vi "Multiple Chassis Synchronization - Scopes Synchronized without TCLK.vi"() -> ()   [LabVIEW 2026]
uses:
  SubVIs/NI SYNC Abstraction/Lib/Clock Routing.ctl
  <instrlib>/niScope/Controls/niScope export destinations.ctl
  SubVIs/NI SYNC Abstraction/Lib/Trigger Routing.ctl
  Types/MyState.ctl
  <instrlib>/niScope/Controls/niScope input clock source.ctl
  Types/MyVariables.ctl
  <instrlib>/niScope/Controls/niScope exportable signals.ctl
  <instrlib>/niFgen/niFgen.llb/niFgen Output Mode.ctl
  <instrlib>/niScope/Configure/Trigger/niScope Configure Trigger Edge.vi
  <instrlib>/niScope/Configure/Trigger/niScope Configure Trigger Digital.vi
  <instrlib>/niSync/niSync.llb/niSync Initialize (IVI).vi
  SubVIs/NI SYNC Abstraction/Lib/Connect Clock Terminals-Array.vi
  SubVIs/NI SYNC Abstraction/Lib/Connect Clock Terminals.vi
  SubVIs/NI SYNC Abstraction/Lib/Connect Trigger Terminals.vi
  <instrlib>/niScope/Acquire/Fetch/niScope Fetch Cluster.vi
  SubVIs/NI SYNC Abstraction/Lib/Disonnect Trigger Terminals.vi
  SubVIs/NI SYNC Abstraction/Lib/Disconnect Clock Terminals-Array.vi
  SubVIs/NI SYNC Abstraction/Lib/Disconnect Clock Terminals.vi
panel:
  in  "Tab Control":T1(tab)
  in  "Master.Scope":refnum<k15>="PXI1_SCOPE1"
  in  "Rest.Scopes":refnum<k15>[](array[refnum])=["PXI2_SCOPE2"]
  in  "Master.6674T_1":refnum<k15>="PXI1_MasterSync"
  in  "Rest.6674T_1":refnum<k15>="PXI2_SlaveSync"
  in  "FGEN.Ref":refnum<k15>="PXI1_FGEN1"
  in  "Routing":enum32{"Clock Routing", "Reference Trigger"}(tab)
  in  "Rest.In --> Clk10":T2={"Source Terminal"="ClkIn", "Destination Terminal"="PXI_Clk10_In"}
  in  "Master.In --> Clk10":T2={"Source Terminal"="ClkIn", "Destination Terminal"="PXI_Clk10_In"}
  in  "Master.Clock --> Out":T2={"Source Terminal"="Oscillator", "Destination Terminal"="ClkOut"}
  in  "Rest.Ref Trigger Source":T3="VAL_RTSI_0"
  in  "Rest.PFI --> Ref Trigger":T4={"Source"="PFI0", "Destination"="PXI_Trig0", "Synchronization Clock"="SyncClkAsync"}
  in  "Master.Ref Trigger --> PFI":T4={"Source"="PXI_Trig0", "Destination"="PFI0", "Synchronization Clock"="SyncClkAsync"}
  in  "Master.Ref Trigger Export":T3="VAL_RTSI_0"
  out "Waveform Graph":T5(graph)
  out "Sample Offset":dbl
  out "error out":errorcluster
  out "Offset Time (s)":dbl format="%#_p"
  # "Scope"
  # "Sync"
  # "Master"
  # "Ref Trigger Export"
  # "None"
  # "None"
  # "None"
  # "Sync"
  # "Scope"
  # "Rest"
  # "Ref Trigger Source"
  # "None"
  # "None"
  # "None"
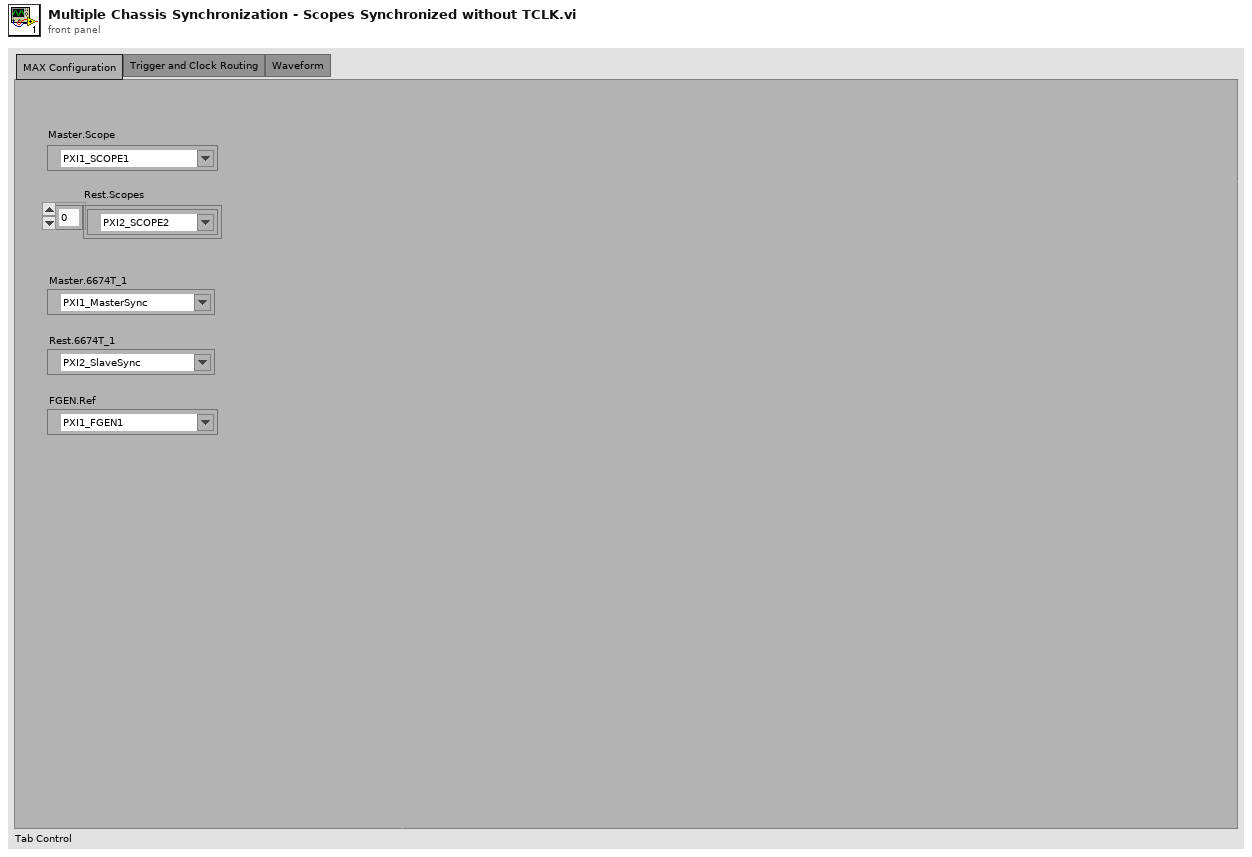
[diagram p1: front panel]
types:
  T1 = enum32{"MAX Configuration", "Trigger and Clock Routing", "Waveform"}
  T2 = typedef "Clock Routing.ctl" = cluster{"Source Terminal":string, "Destination Terminal":string}
  T3 = typedef "niScope export destinations.ctl" = string
  T4 = typedef "Trigger Routing.ctl" = cluster{"Source":string, "Destination":string, "Synchronization Clock":string}
  T5 = cluster{"relativeInitialX":dbl, "xIncrement":dbl, "wfm":dbl[]}[]
  T6 = typedef "niScope input clock source.ctl" = u16
  T7 = typedef "MyState.ctl" = enum16{"Initialize", "SCOPE: Config.Master", "SCOPE: Config.Rest", "SYNC: Device.Init", "SYNC: ConnectClock.Master", "SYNC: ConnectClock.Rest", "SYNC: ConnectSyncPulse.Master", "SYNC: ConnectSyncPulse.Rest", "SYNC: ConnectRefTrigger.Master", "SYNC: ConnectRefTrigger.Rest", "TCLK: Config.Master", "TCLK: Config.Rest", "TCLK: ApplyManualCalibration", "TCLK: SendSyncPulse", "SYNC: DisconnectSyncPulse.Master", "SYNC: DisconnectSyncPulse.Rest", "SYNC: ConnectStartTrigger.Master", "SYNC: ConnectStartTrigger.Rest", "TCLK: Commit", "FGEN: StartSquareWave", "SCOPE: Acquire", "FGEN: StopSquareWave", "SYNC: DisconnectStartTrigger.Master", "SYNC: DisconnectStartTrigger.Rest", "SYNC: DisconnectRefTrigger.Master", "SYNC: DisconnectRefTrigger.Rest", "SYNC: DisconnectClock.Master", "SYNC: DisconnectClock.Rest", "Shutdown"}
  T8 = typedef "MyVariables.ctl" = cluster{"Master":cluster{"TimeSync.Ref":refnum<k15>, "TCLK.Ref":refnum<k20>, "Clock":cluster{"Clock --> Out":T2, "In --> Clk10":T2}, "Sync Pulse":cluster{"Sync Pulse Export":string, "Sync Pulse Export --> PFI":T4, "PFI --> Sync Pulse Source":T4, "Sync Pulse Source":string}, "Start Trigger":cluster{"Start Trigger Export":T3, "Start Trigger --> PFI":T4}, "Scope.Ref":refnum<k15>, "Ref Trigger":cluster{"Ref Trigger Export":T3, "Ref Trigger --> PFI":T4}}, "Rest":cluster{"TimeSync.Ref":refnum<k15>, "TCLK.Refs":refnum<k20>[], "Clock":cluster{"In --> Clk10":T2}, "Sync Pulse":cluster{"PFI --> Sync Pulse Source":T4, "Sync Pulse Source":string}, "Start Trigger":cluster{"PFI --> Start Trigger":T4, "Start Trigger Source":T3}, "Scope.Refs":refnum<k15>[], "Ref Trigger":cluster{"PFI --> Ref Trigger":T4, "Ref Trigger Source":T3}}, "FGEN.Ref":refnum<k15>}
  T9 = typedef "niScope exportable signals.ctl" = u16
  T10 = typedef "niFgen Output Mode.ctl" = u32
  T11 = cluster{"relativeInitialX":dbl, "xIncrement":dbl, "wfm":dbl[]}
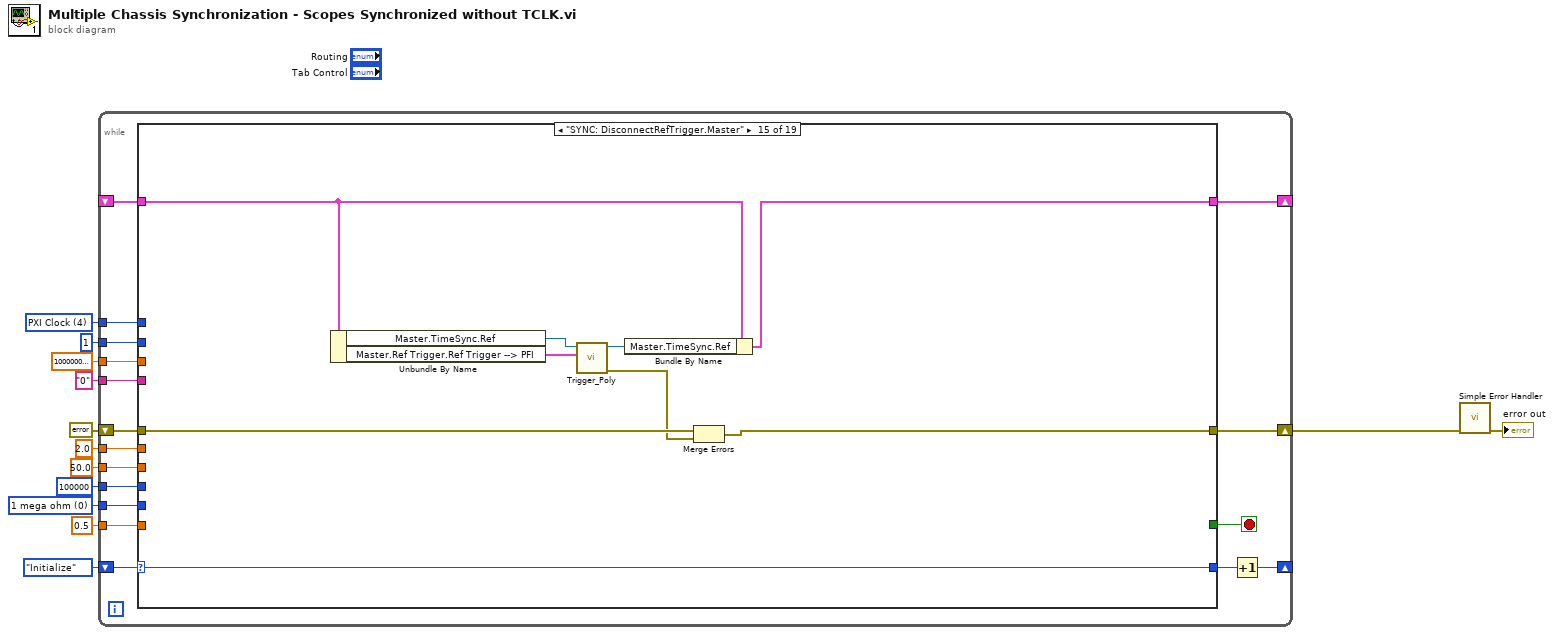
[diagram p0: block diagram]
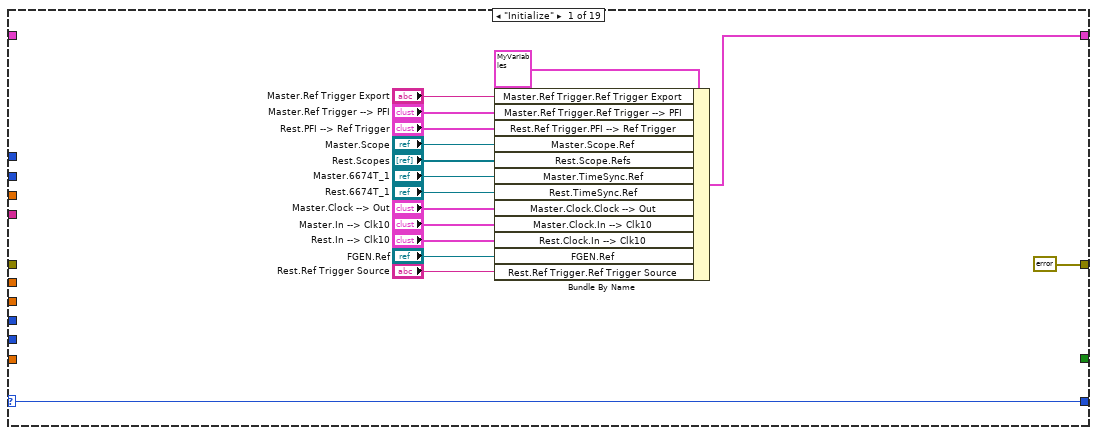
[diagram p2: hidden frame]
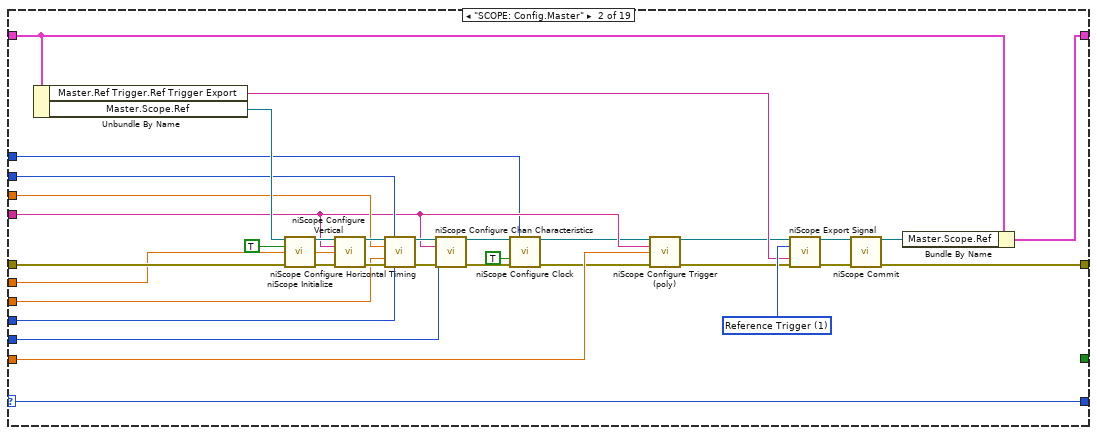
[diagram p3: hidden frame]
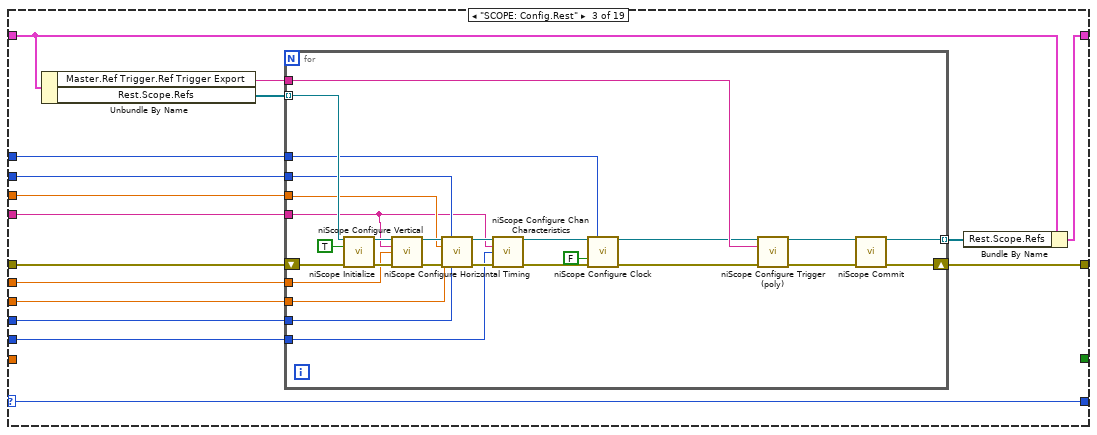
[diagram p4: hidden frame]
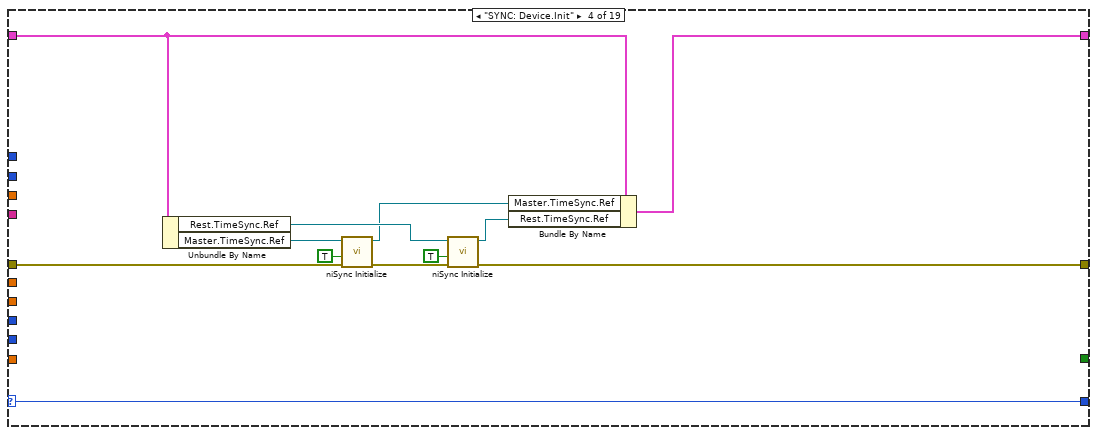
[diagram p5: hidden frame]
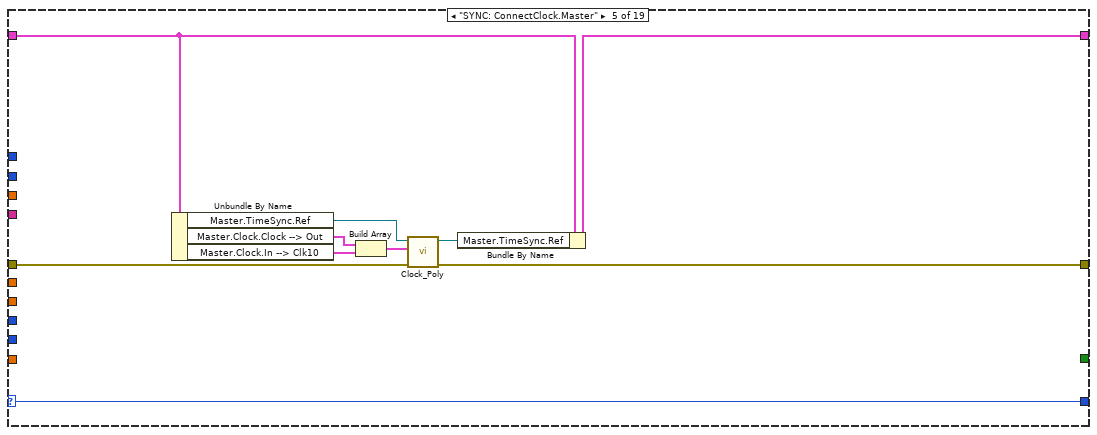
[diagram p6: hidden frame]
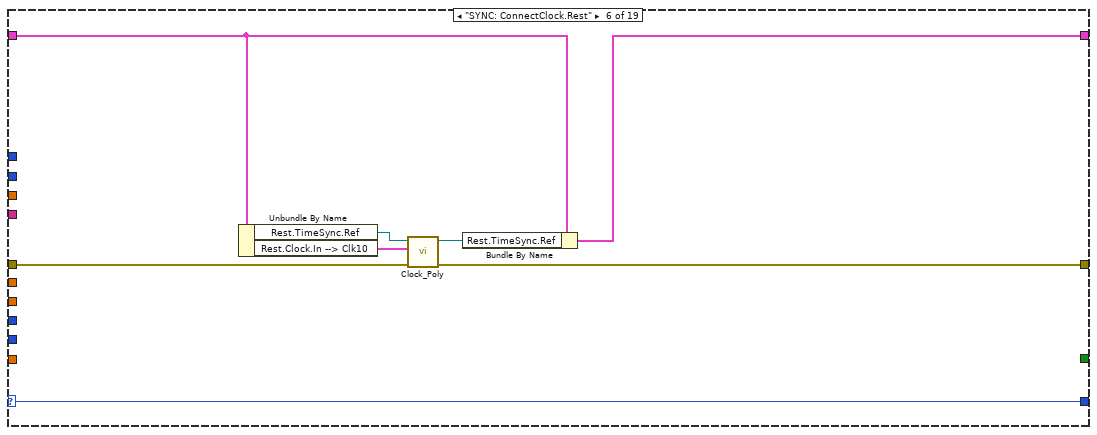
[diagram p7: hidden frame]
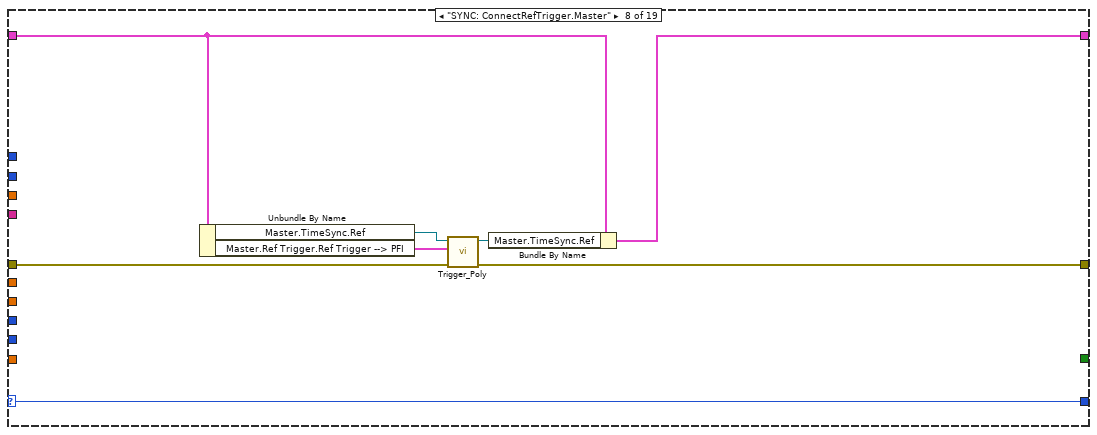
[diagram p9: hidden frame]
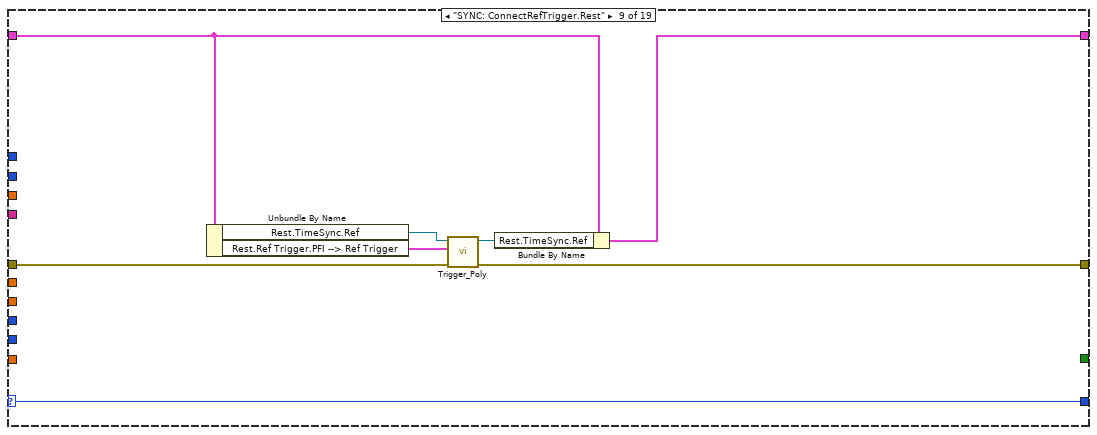
[diagram p10: hidden frame]
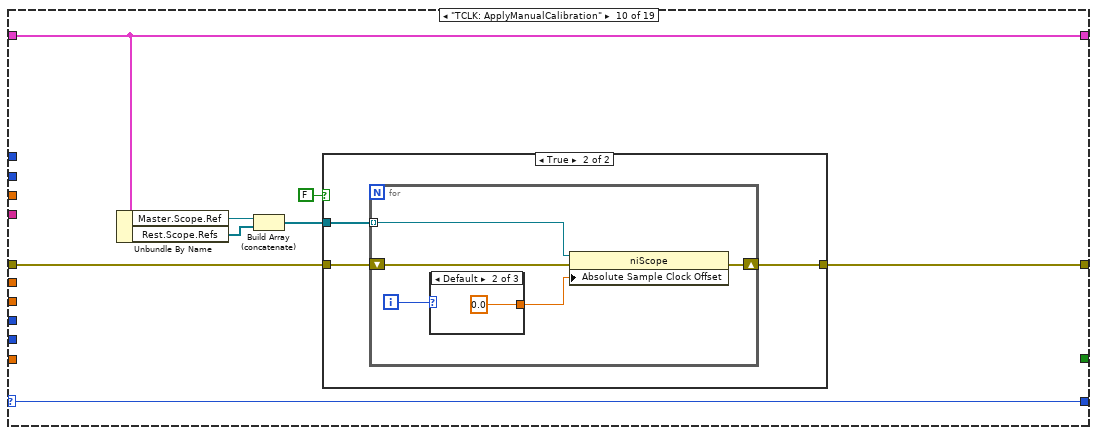
[diagram p11: hidden frame]
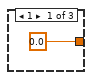
[diagram p13: hidden frame]
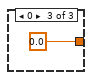
[diagram p14: hidden frame]
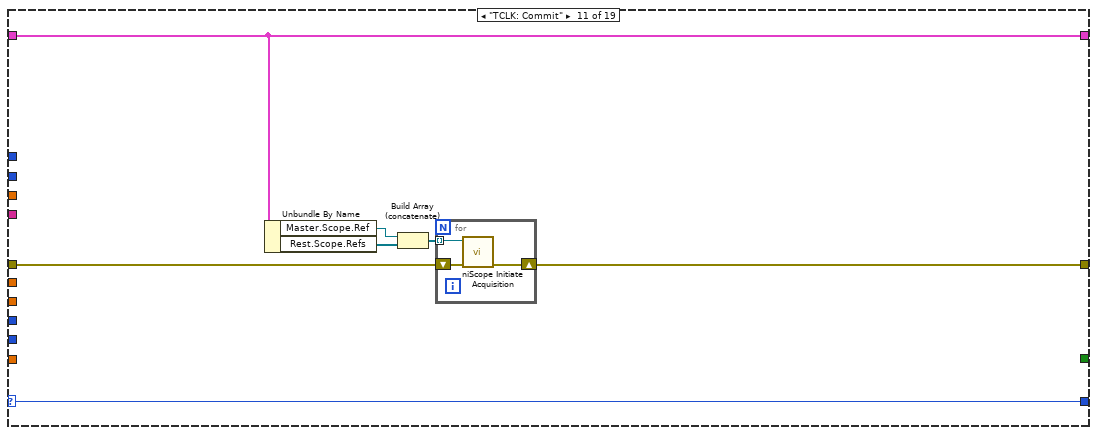
[diagram p15: hidden frame]
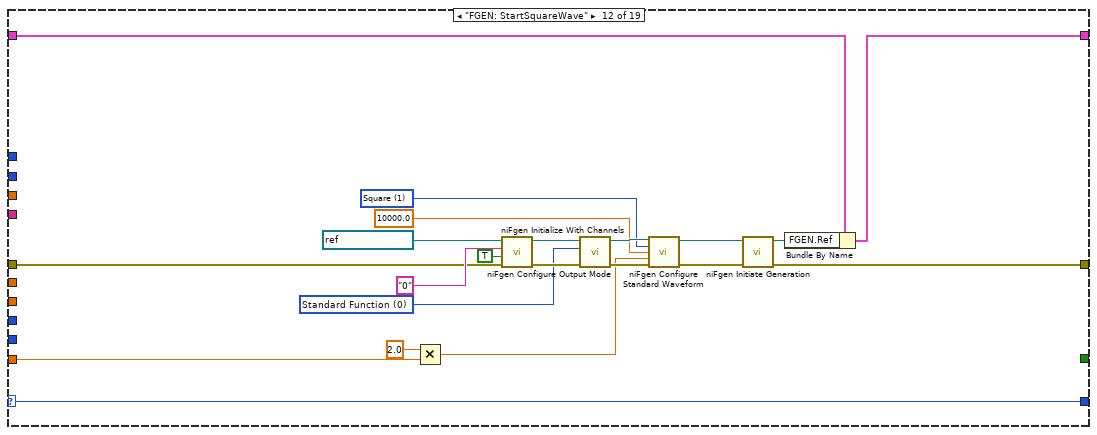
[diagram p16: hidden frame]
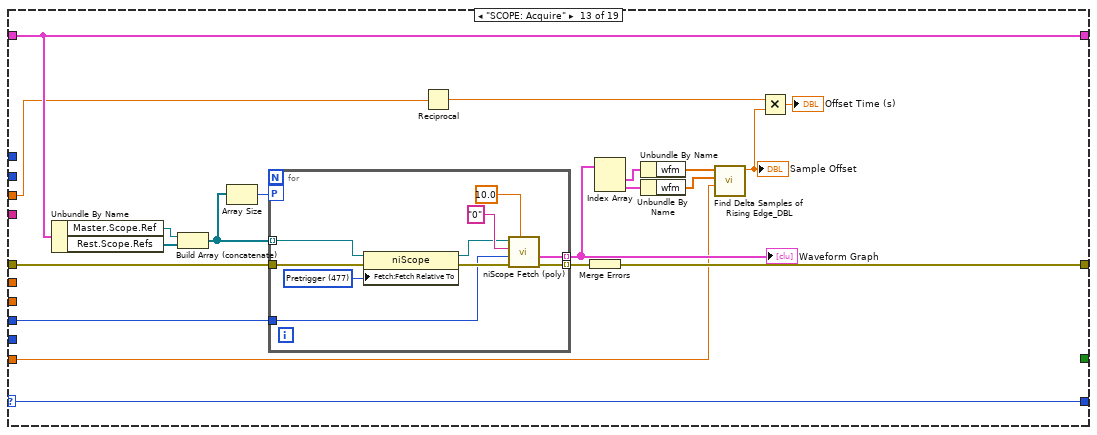
[diagram p17: hidden frame]
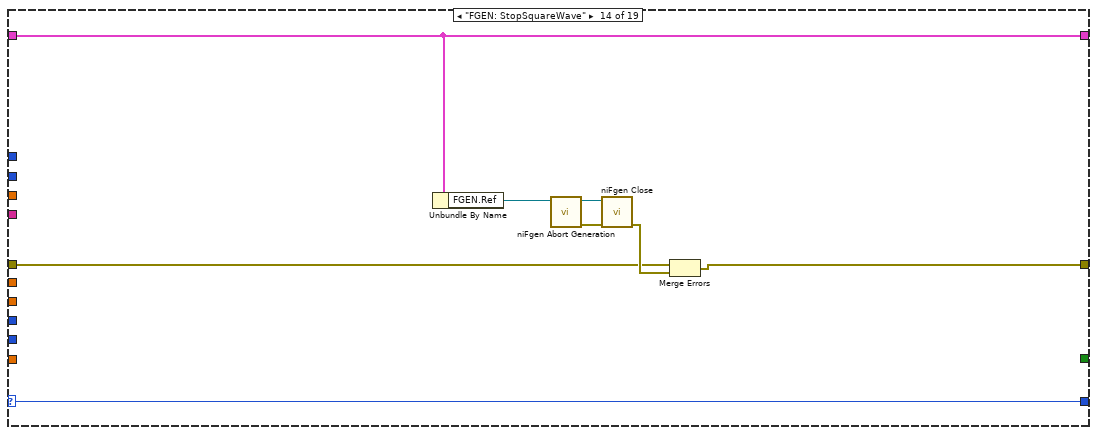
[diagram p18: hidden frame]
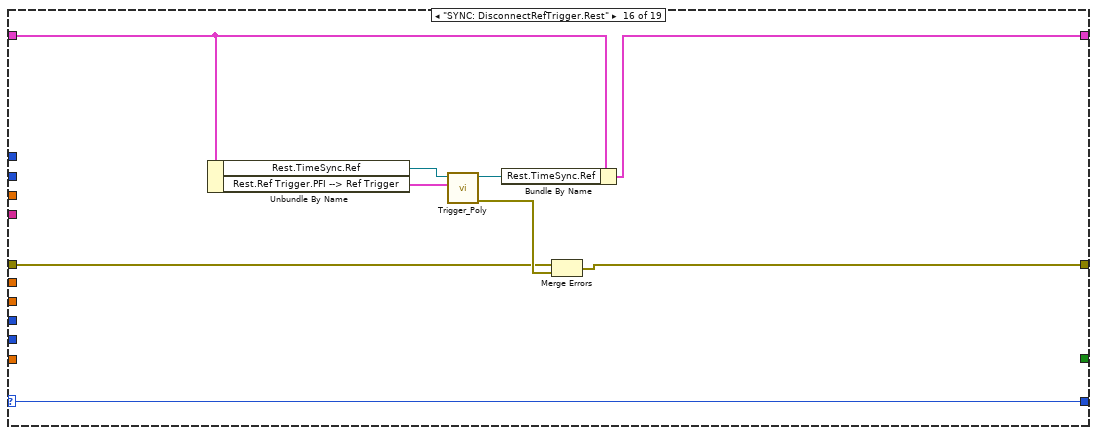
[diagram p19: hidden frame]
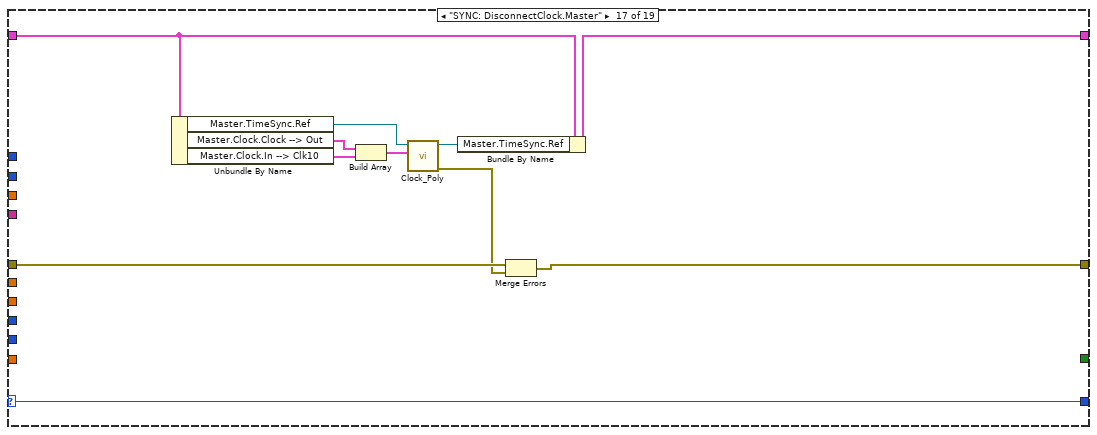
[diagram p20: hidden frame]
diagram:
  w1 = T6 4 items=["None"=0, "RTSI Clock"=1, "PFI 0"=6, "PFI 1"=2, "PFI 2"=3, "PXI Clock"=4, "External"=5, "Clock In"=7] ("input clock source")
  w5 = u32 0 items=["1 mega ohm"=0, "50 ohms"=2] ("input impedance")
  n1 = while {
    shift-right: [w23] -> _
    shift-left: MyState."Initialize" -> [w30]
    shift-right: [w29] -> _
    shift-left: _ -> [w28]
    shift-right: [w26] -> w11
    shift-left: errorcluster {"status"=FALSE, "code"=0, "source"=""} ("error out") -> [w27]
    tunnel: 100000000.0 ("min sample rate") -> [w22]
    tunnel: 100000 ("min record length") -> [w21]
    tunnel: 2.0 ("vertical offset") -> [w20]
    tunnel: 50.0 ("reference position") -> [w19]
    tunnel: w5 -> [w18]
    tunnel: 1 ("number of records") -> [w17]
    tunnel: "0" ("channels") -> [w16]
    tunnel: 0.5 ("trigger level") -> [w15]
    tunnel: w1 -> [w14]
    stop <- w24 stop-if-true
    n2 = case shown="\"SYNC: DisconnectRefTrigger.Master\"" w30 {
      selector: w30 -> [w39 w80 w96 w125 w136 w147 w156 w158 w166 w180 w199 w210 w243 w254 w266 w275 w283 w295 w301]
      tunnel: [w40 w79 w95 w129 w144 w152 w154 w163 w171 w179 w196 w207 w240 w259 w269 w278 w289 w298 w312] -> w29
      tunnel: w28 -> [_ w70 w92 w130 w145 w153 w154 w164 w172 w179 w196 w209 w240 w259 w270 w279 w290 w299 w312]
      tunnel: [w39 w80 w96 w125 w136 w147 w156 w158 w166 w180 w199 w210 w243 w254 w266 w275 w283 w295 w301] -> w25
      tunnel: [errorcluster {"status"=FALSE, "code"=0, "source"=""} ("error out") w56 w94 w126 w141 w149 w155 w160 w168 w174 w194 w211 w237 w255 w262 w272 w281 w292 w302] -> w26
      tunnel: w27 -> [_ w71 w93 w124 w137 w148 w155 w159 w167 w175 w195 w212 w242 w256 w264 w271 w282 w293 w305]
      tunnel: [_ _ _ _ _ _ _ _ _ _ _ _ _ _ _ _ _ _ TRUE] -> w24
      tunnel: w22 -> [_ w64 w87 _ _ _ _ _ _ _ _ _ w228 _ _ _ _ _ _]
      tunnel: w21 -> [_ w63 w83 _ _ _ _ _ _ _ _ _ w229 _ _ _ _ _ _]
      tunnel: w20 -> [_ w62 w85 _ _ _ _ _ _ _ _ _ _ _ _ _ _ _ _]
      tunnel: w19 -> [_ w61 w84 _ _ _ _ _ _ _ _ _ _ _ _ _ _ _ _]
      tunnel: w18 -> [_ w60 w82 _ _ _ _ _ _ _ _ _ _ _ _ _ _ _ _]
      tunnel: w17 -> [_ w59 w88 _ _ _ _ _ _ _ _ _ _ _ _ _ _ _ _]
      tunnel: w16 -> [_ w58 w86 _ _ _ _ _ _ _ _ _ _ _ _ _ _ _ _]
      tunnel: w15 -> [_ w57 _ _ _ _ _ _ _ _ _ w205 w224 _ _ _ _ _ _]
      tunnel: w14 -> [_ w47 w81 _ _ _ _ _ _ _ _ _ _ _ _ _ _ _ _]
      frame "Initialize" {
        n3 = Bundle By Name(cluster=T8 {"Master"={"TimeSync.Ref"="PXI_Trig0", "TCLK.Ref"=refnum, "Clock"={"Clock --> Out"={"Source Terminal"="Oscillator", "Destination Terminal"="ClkOut"}, "In --> Clk10"={"Source Terminal"="ClkIn", "Destination Terminal"="PXI_Clk10_In"}}, "Sync Pulse"={"Sync Pulse Export"="SyncClkFullSpeed", "Sync Pulse Export --> PFI"={"Source"="ClkIn", "Destination"="PXI_Clk10_In", "Synchronization Clock"="SyncClkAsync"}, "PFI --> Sync Pulse Source"={"Source"="PXI_Trig2", "Destination"="PFI2", "Synchronization Clock"="SyncClkAsync"}, "Sync Pulse Source"="PFI1"}, "Start Trigger"={"Start Trigger Export"="PXI_Trig2", "Start Trigger --> PFI"={"Source"="SyncClkAsync", "Destination"="VAL_RTSI_2", "Synchronization Clock"=""}}, "Scope.Ref"="", "Ref Trigger"={"Ref Trigger Export"="VAL_RTSI_2", "Ref Trigger --> PFI"={"Source"="PXI_Trig3", "Destination"="PFI0", "Synchronization Clock"="SyncClkAsync"}}}, "Rest"={"TimeSync.Ref"="", "TCLK.Refs"=[], "Clock"={"In --> Clk10"={"Source Terminal"="PXI_Trig0", "Destination Terminal"="PFI2"}}, "Sync Pulse"={"PFI --> Sync Pulse Source"={"Source"="PFI1", "Destination"="PXI_Trig1", "Synchronization Clock"="SyncClkAsync"}, "Sync Pulse Source"="PXI_Trig1"}, "Start Trigger"={"PFI --> Start Trigger"={"Source"="PFI1", "Destination"="PXI_Trig2", "Synchronization Clock"="SyncClkAsync"}, "Start Trigger Source"="VAL_RTSI_2"}, "Scope.Refs"=[], "Ref Trigger"={"PFI --> Ref Trigger"={"Source"="PFI0", "Destination"="PXI_Trig3", "Synchronization Clock"="SyncClkAsync"}, "Ref Trigger Source"="VAL_RTSI_3"}}, "FGEN.Ref"=""} ("Routes"), "Master.Ref Trigger.Ref Trigger Export"="Master.Ref Trigger Export", "Master.Ref Trigger.Ref Trigger --> PFI"="Master.Ref Trigger --> PFI", "Rest.Ref Trigger.PFI --> Ref Trigger"="Rest.PFI --> Ref Trigger", "Master.Scope.Ref"="Master.Scope", "Rest.Scope.Refs"="Rest.Scopes", "Master.TimeSync.Ref"="Master.6674T_1", "Rest.TimeSync.Ref"="Rest.6674T_1", "Master.Clock.Clock --> Out"="Master.Clock --> Out", "Master.Clock.In --> Clk10"="Master.In --> Clk10", "Rest.Clock.In --> Clk10"="Rest.In --> Clk10", "FGEN.Ref"="FGEN.Ref", "Rest.Ref Trigger.Ref Trigger Source"="Rest.Ref Trigger Source") -> (w40:T8)
      }
      frame "SCOPE: Config.Master" {
        w66 = T9 1 items=["None"=0, "Start Trigger"=2, "Advance Trigger"=5, "Reference Trigger"=1, "End of Record Event"=4, "End of Acquisition Event"=3, "Ready for Start Event"=7, "Ready for Advance Event"=6, "Ready for Reference Event"=10, "Reference Clock"=100, "Sample Clock"=101, "5 Volt Power"=13] ("signal")
        n4 = Unbundle By Name(w70) -> ("Master.Ref Trigger.Ref Trigger Export"=w65:T3, "Master.Scope.Ref"=w69:refnum<k15>)
        n5 = call <instrlib>:"niScope Initialize.vi"("resource name"=w69, "id query"=TRUE, "error in"=w71) -> ("instrument handle"=w77:refnum<k15>, "error out"=w74:errorcluster)  [unwired: 11 in]
        n6 = call <instrlib>:"niScope Configure Vertical.vi"("instrument handle"=w77, "channels"=w58, "vertical range"=w62, "error in"=w74) -> ("instrument handle out"=w76:refnum<k15>, "error out"=w73:errorcluster)  [unwired: 10 in]
        n7 = call <instrlib>:"niScope Configure Horizontal Timing.vi"("instrument handle"=w76, "number of records"=w59, "min sample rate"=w64, "reference position"=w61, "error in"=w73, "min record length"=w63) -> ("instrument handle out"=w75:refnum<k15>, "error out"=w72:errorcluster)  [unwired: 8 in]
        n8 = call <instrlib>:"niScope Configure Chan Characteristics.vi"("instrument handle"=w75, "channels"=w58, "input impedance"=w60, "error in"=w72) -> ("instrument handle out"=w49:refnum<k15>, "error out"=w51:errorcluster)  [unwired: 10 in]
        n9 = call <instrlib>:"niScope Configure Clock.vi"("instrument handle"=w49, "input clock source"=w47, "master enabled"=TRUE, "error in"=w51) -> ("instrument handle out"=w48:refnum<k15>, "error out"=w50:errorcluster)  [unwired: 10 in]
        n10 = call-poly <instrlib>:"niScope Configure Trigger (poly).vi"("instrument handle"=w48, "trigger source"=w58, "trigger level"=w57, "error in"=w50) -> ("instrument handle out"=w53:refnum<k15>, "error out"=w54:errorcluster)  [unwired: 10 in]
        n11 = call <instrlib>:"niScope Export Signal.vi"("instrument handle"=w53, "signal"=w66, "output terminal"=w65, "error in"=w54) -> ("instrument handle out"=w67:refnum<k15>, "error out"=w68:errorcluster)  [unwired: 10 in]
        n12 = call <instrlib>:"niScope Commit.vi"("instrument handle"=w67, "error in"=w68) -> ("instrument handle out"=w55:refnum<k15>, "error out"=w56:errorcluster)  [unwired: 12 in]
        n13 = Bundle By Name(cluster=w70, "Master.Scope.Ref"=w55) -> (w79:T8)
      }
      frame "SCOPE: Config.Rest" {
        n14 = Unbundle By Name(w92) -> ("Master.Ref Trigger.Ref Trigger Export"=w89:T3, "Rest.Scope.Refs"=w90:refnum<k15>[])
        n15 = for {
          shift-right: [w104] -> w94
          shift-left: w93 -> [w116]
          tunnel: [w103] -> w91 mode=indexing
          tunnel: w90 -> [w113] mode=indexing
          tunnel: w89 -> [w112]
          tunnel: w88 -> [w111]
          tunnel: w87 -> [w110]
          tunnel: w86 -> [w109]
          tunnel: w85 -> [w108]
          tunnel: w84 -> [w107]
          tunnel: w83 -> [w106]
          tunnel: w82 -> [w105]
          tunnel: w81 -> [w97]
          n16 = call <instrlib>:"niScope Initialize.vi"("resource name"=w113, "id query"=TRUE, "error in"=w116) -> ("instrument handle"=w122:refnum<k15>, "error out"=w119:errorcluster)  [unwired: 11 in]
          n17 = call <instrlib>:"niScope Configure Vertical.vi"("instrument handle"=w122, "channels"=w109, "vertical range"=w108, "error in"=w119) -> ("instrument handle out"=w121:refnum<k15>, "error out"=w118:errorcluster)  [unwired: 10 in]
          n18 = call <instrlib>:"niScope Configure Horizontal Timing.vi"("instrument handle"=w121, "number of records"=w111, "min sample rate"=w110, "reference position"=w107, "error in"=w118, "min record length"=w106) -> ("instrument handle out"=w120:refnum<k15>, "error out"=w117:errorcluster)  [unwired: 8 in]
          n19 = call <instrlib>:"niScope Configure Chan Characteristics.vi"("instrument handle"=w120, "channels"=w109, "input impedance"=w105, "error in"=w117) -> ("instrument handle out"=w101:refnum<k15>, "error out"=w99:errorcluster)  [unwired: 10 in]
          n20 = call <instrlib>:"niScope Configure Clock.vi"("instrument handle"=w101, "input clock source"=w97, "master enabled"=FALSE, "error in"=w99) -> ("instrument handle out"=w100:refnum<k15>, "error out"=w98:errorcluster)  [unwired: 10 in]
          n21 = call-poly <instrlib>:"niScope Configure Trigger (poly).vi"("instrument handle"=w100, "trigger source"=w112, "error in"=w98) -> ("instrument handle out"=w114:refnum<k15>, "error out"=w115:errorcluster)  [unwired: 11 in]
          n22 = call <instrlib>:"niScope Commit.vi"("instrument handle"=w114, "error in"=w115) -> ("instrument handle out"=w103:refnum<k15>, "error out"=w104:errorcluster)  [unwired: 12 in]
        }
        n23 = Bundle By Name(cluster=w92, "Rest.Scope.Refs"=w91) -> (w95:T8)
      }
      frame "SYNC: Device.Init" {
        n24 = Unbundle By Name(w130) -> ("Rest.TimeSync.Ref"=w134:refnum<k15>, "Master.TimeSync.Ref"=w135:refnum<k15>)
        n25 = call-poly <instrlib>:"niSync Initialize.vi"("error in (no error)"=w124, "reset device (F)"=TRUE, "resource name"=w135) -> ("error out"=w133:errorcluster, "instrument handle out"=w128:refnum<k15>)  [unwired: 7 in]
        n26 = call-poly <instrlib>:"niSync Initialize.vi"("error in (no error)"=w133, "reset device (F)"=TRUE, "resource name"=w134) -> ("error out"=w126:errorcluster, "instrument handle out"=w127:refnum<k15>)  [unwired: 7 in]
        n27 = Bundle By Name(cluster=w130, "Master.TimeSync.Ref"=w128, "Rest.TimeSync.Ref"=w127) -> (w129:T8)
      }
      frame "SYNC: ConnectClock.Master" {
        n28 = Unbundle By Name(w145) -> ("Master.TimeSync.Ref"=w143:refnum<k15>, "Master.Clock.Clock --> Out"=w140:T2, "Master.Clock.In --> Clk10"=w139:T2)
        n29 = Build Array(w140, w139) -> (w138:T2[])
        n30 = call-poly "Clock_Poly.vi"("error in (no error)"=w137, "Clock Routing"=w138, "instrument handle"=w143) -> ("error out"=w141:errorcluster, "instrument handle out"=w142:refnum<k15>)  [unwired: 7 in]
        n31 = Bundle By Name(cluster=w145, "Master.TimeSync.Ref"=w142) -> (w144:T8)
      }
      frame "SYNC: ConnectClock.Rest" {
        n32 = Unbundle By Name(w153) -> ("Rest.TimeSync.Ref"=w151:refnum<k15>, "Rest.Clock.In --> Clk10"=w146:T2)
        n33 = call-poly "Clock_Poly.vi"("error in (no error)"=w148, "Clock Routing"=w146, "instrument handle"=w151) -> ("error out"=w149:errorcluster, "instrument handle out"=w150:refnum<k15>)  [unwired: 7 in]
        n34 = Bundle By Name(cluster=w153, "Rest.TimeSync.Ref"=w150) -> (w152:T8)
      }
      frame Default {
      }
      frame "SYNC: ConnectRefTrigger.Master" {
        n35 = Unbundle By Name(w164) -> ("Master.TimeSync.Ref"=w162:refnum<k15>, "Master.Ref Trigger.Ref Trigger --> PFI"=w157:T4)
        n36 = call-poly "Trigger_Poly.vi"("error in (no error)"=w159, "Routing Information"=w157, "instrument handle"=w162) -> ("error out"=w160:errorcluster, "instrument handle out"=w161:refnum<k15>)  [unwired: 7 in]
        n37 = Bundle By Name(cluster=w164, "Master.TimeSync.Ref"=w161) -> (w163:T8)
      }
      frame "SYNC: ConnectRefTrigger.Rest" {
        n38 = Unbundle By Name(w172) -> ("Rest.TimeSync.Ref"=w170:refnum<k15>, "Rest.Ref Trigger.PFI --> Ref Trigger"=w165:T4)
        n39 = call-poly "Trigger_Poly.vi"("error in (no error)"=w167, "Routing Information"=w165, "instrument handle"=w170) -> ("error out"=w168:errorcluster, "instrument handle out"=w169:refnum<k15>)  [unwired: 7 in]
        n40 = Bundle By Name(cluster=w172, "Rest.TimeSync.Ref"=w169) -> (w171:T8)
      }
      frame "TCLK: ApplyManualCalibration" {
        n41 = Unbundle By Name(w179) -> ("Master.Scope.Ref"=w177:refnum<k15>, "Rest.Scope.Refs"=w176:refnum<k15>[])
        n42 = Build Array (concatenate)(w177, w176) -> (w173:refnum<k15>[])
        n43 = case shown="True" FALSE {
          tunnel: w175 -> [w181 w183]
          tunnel: [w181 w182] -> w174
          tunnel: w173 -> [_ w184]
          frame False {
          }
          frame True {
            n44 = for {
              tunnel: w184 -> [w186] mode=indexing
              shift-right: [w187] -> w182
              shift-left: w183 -> [w188]
              i -> [w189]
              n45 = case shown="Default" w189 {
                tunnel: [0.0 ("delay") 0.0 ("delay") 0.0 ("delay")] -> w185
                frame 1 {
                }
                frame Default {
                }
                frame 0 {
                }
              }
              n46 = property class="niScope"(reference=w186, error in=w188, "Absolute Sample Clock Offset"=w185) -> (error out=w187:errorcluster)  [unwired: 1 out]
            }
          }
        }
      }
      frame "TCLK: Commit" {
        n47 = Unbundle By Name(w196) -> ("Master.Scope.Ref"=w198:refnum<k15>, "Rest.Scope.Refs"=w197:refnum<k15>[])
        n48 = Build Array (concatenate)(w198, w197) -> (w193:refnum<k15>[])
        n49 = for {
          shift-right: [w201] -> w194
          shift-left: w195 -> [w202]
          tunnel: w193 -> [w200] mode=indexing
          n50 = call <instrlib>:"niScope Initiate Acquisition.vi"("instrument handle"=w200, "error in"=w202) -> ("error out"=w201:errorcluster)  [unwired: 12 in, 1 out]
        }
      }
      frame "FGEN: StartSquareWave" {
        w215 = u16 1 items=["Sine", "Square", "Triangle", "Ramp Up", "Ramp Down", "DC", "Noise"] ("Standard Waveform")
        w213 = T10 0 items=["Standard Function", "Frequency List", "Arbitrary Waveform", "Arbitrary Sequence", "Script"] ("output mode")
        n51 = Multiply(x=2.0, y=w205) -> (x*y=w204:dbl)
        n52 = call <instrlib>:"niFgen Initialize With Channels.vi"("error in (no error)"=w212, "Reset Device (default: False)"=TRUE, "Channel Name"="0", "Resource Name"=refnum<k15> "PXI1_FGEN1" ("FGEN Resource Name")) -> ("error out"=w223:errorcluster, "Instrument Handle Out"=w222:refnum<k15>)  [unwired: 6 in]
        n53 = call <instrlib>:"niFgen Configure Output Mode.vi"("error in (no error)"=w223, "Output Mode (default: 0=Standard Function)"=w213, "Instrument Handle"=w222) -> ("error out"=w221:errorcluster, "Instrument Handle Out"=w220:refnum<k15>)  [unwired: 6 in]
        n54 = call <instrlib>:"niFgen Configure Standard Waveform.vi"("Instrument Handle"=w220, "Waveform"=w215, "Frequency"=10000.0, "Amplitude"=w204, "error in (no error)"=w221) -> ("Instrument Handle Out"=w219:refnum<k15>, "error out"=w218:errorcluster)  [unwired: 9 in]
        n55 = call <instrlib>:"niFgen Initiate Generation.vi"("error in (no error)"=w218, "Instrument Handle"=w219) -> ("error out"=w211:errorcluster, "Instrument Handle Out"=w208:refnum<k15>)  [unwired: 8 in]
        n56 = Bundle By Name(cluster=w209, "FGEN.Ref"=w208) -> (w207:T8)
      }
      frame "SCOPE: Acquire" {
        n57 = Unbundle By Name(w240) -> ("Master.Scope.Ref"=w238:refnum<k15>, "Rest.Scope.Refs"=w239:refnum<k15>[])
        n58 = Build Array (concatenate)(w238, w239) -> (w236:refnum<k15>[])
        n59 = Array Size(array=w236) -> (size(s)=w235:i32)
        n60 = for {
          tunnel: w236 -> [w250] mode=indexing
          tunnel: [w245] -> w230 mode=indexing
          tunnel: w242 -> [w249]
          tunnel: [w253] -> w241 mode=indexing
          workers-P: w235 -> [_]
          tunnel: w229 -> [w244]
          w246 = 477 items=["Start"=482, "Trigger"=483, "Pretrigger"=477, "Now"=481, "Read Pointer"=388] ("Fetch:Fetch Relative To")
          n61 = property class="niScope"(reference=w250, error in=w249, "Fetch:Fetch Relative To"=w246) -> (reference out=w247:refnum<k15>, error out=w248:errorcluster)
          n62 = call-poly <instrlib>:"niScope Fetch (poly).vi"("timeout"=10.0, "error in"=w248, "numSamples"=w244, "channels"="0", "instrument handle"=w247) -> ("error out"=w253:errorcluster, "waveform"=w245:T11)  [unwired: 3 in, 2 out]
        }
        "Waveform Graph" <- w230
        n63 = Reciprocal(x=w228) -> (1/x=w226:dbl)
        n64 = Merge Errors(w241) -> (w237:errorcluster)
        n65 = Index Array(array=w230) -> (element #1=w234:T11, element #2=w233:T11)  [unwired: 2 in]
        n66 = Unbundle By Name(w234) -> ("wfm"=w231:dbl[])
        n67 = Unbundle By Name(w233) -> ("wfm"=w232:dbl[])
        n68 = call "Find Delta Samples of Rising Edge_DBL.vi"("Trigger Level"=w224, "Channel 2"=w232, "Channel 1"=w231) -> ("Sample Offset"=w227:dbl)  [unwired: 8 in]
        "Sample Offset" <- w227
        n69 = Multiply(x=w226, y=w227) -> (x*y=→"Offset Time (s)":dbl)
      }
      frame "FGEN: StopSquareWave" {
        n70 = Unbundle By Name(w259) -> ("FGEN.Ref"=w258:refnum<k15>)
        n71 = call <instrlib>:"niFgen Abort Generation.vi"("Instrument Handle"=w258) -> ("error out"=w261:errorcluster, "Instrument Handle Out"=w260:refnum<k15>)  [unwired: 9 in]
        n72 = call <instrlib>:"niFgen Close.vi"("error in (no error)"=w261, "Instrument Handle"=w260) -> ("error out"=w257:errorcluster)  [unwired: 9 in]
        n73 = Merge Errors(w256, w257) -> (w255:errorcluster)
      }
      frame "SYNC: DisconnectRefTrigger.Master" {
        n74 = Unbundle By Name(w270) -> ("Master.TimeSync.Ref"=w268:refnum<k15>, "Master.Ref Trigger.Ref Trigger --> PFI"=w265:T4)
        n75 = call-poly "Trigger_Poly.vi"("Routing Information"=w265, "instrument handle"=w268) -> ("error out"=w263:errorcluster, "instrument handle out"=w267:refnum<k15>)  [unwired: 8 in]
        n76 = Bundle By Name(cluster=w270, "Master.TimeSync.Ref"=w267) -> (w269:T8)
        n77 = Merge Errors(w264, w263) -> (w262:errorcluster)
      }
      frame "SYNC: DisconnectRefTrigger.Rest" {
        n78 = Unbundle By Name(w279) -> ("Rest.TimeSync.Ref"=w277:refnum<k15>, "Rest.Ref Trigger.PFI --> Ref Trigger"=w274:T4)
        n79 = call-poly "Trigger_Poly.vi"("Routing Information"=w274, "instrument handle"=w277) -> ("error out"=w273:errorcluster, "instrument handle out"=w276:refnum<k15>)  [unwired: 8 in]
        n80 = Bundle By Name(cluster=w279, "Rest.TimeSync.Ref"=w276) -> (w278:T8)
        n81 = Merge Errors(w271, w273) -> (w272:errorcluster)
      }
      frame "SYNC: DisconnectClock.Master" {
        n82 = Unbundle By Name(w290) -> ("Master.TimeSync.Ref"=w288:refnum<k15>, "Master.Clock.Clock --> Out"=w286:T2, "Master.Clock.In --> Clk10"=w285:T2)
        n83 = Build Array(w286, w285) -> (w284:T2[])
        n84 = call-poly "Clock_Poly.vi"("Clock Routing"=w284, "instrument handle"=w288) -> ("error out"=w280:errorcluster, "instrument handle out"=w287:refnum<k15>)  [unwired: 8 in]
        n85 = Bundle By Name(cluster=w290, "Master.TimeSync.Ref"=w287) -> (w289:T8)
        n86 = Merge Errors(w282, w280) -> (w281:errorcluster)
      }
      frame "SYNC: DisconnectClock.Rest" {
        n87 = Unbundle By Name(w299) -> ("Rest.TimeSync.Ref"=w297:refnum<k15>, "Rest.Clock.In --> Clk10"=w294:T2)
        n88 = call-poly "Clock_Poly.vi"("Clock Routing"=w294, "instrument handle"=w297) -> ("error out"=w291:errorcluster, "instrument handle out"=w296:refnum<k15>)  [unwired: 8 in]
        n89 = Bundle By Name(cluster=w299, "Rest.TimeSync.Ref"=w296) -> (w298:T8)
        n90 = Merge Errors(w293, w291) -> (w292:errorcluster)
      }
      frame "Shutdown" {
        n91 = Unbundle By Name(w312) -> ("Master.TimeSync.Ref"=w311:refnum<k15>, "Rest.TimeSync.Ref"=w310:refnum<k15>, "Master.Scope.Ref"=w309:refnum<k15>, "Rest.Scope.Refs"=w308:refnum<k15>[])
        n92 = Build Array(w311, w310) -> (w306:refnum<k15>[])
        n93 = Build Array (concatenate)(w309, w308) -> (w307:refnum<k15>[])
        n94 = for {
          tunnel: w306 -> [w314] mode=indexing
          tunnel: [w313] -> w303 mode=indexing
          n95 = call <instrlib>:"niSync Close.vi"("instrument handle"=w314) -> ("error out"=w313:errorcluster)  [unwired: 10 in]
        }
        n96 = for {
          tunnel: w307 -> [w316] mode=indexing
          tunnel: [w315] -> w304 mode=indexing
          n97 = call <instrlib>:"niScope Close.vi"("instrument handle"=w316) -> ("error out"=w315:errorcluster)  [unwired: 14 in]
        }
        n98 = Merge Errors(w305, w304, w303) -> (w302:errorcluster)
      }
    }
    n99 = Increment(x=w25) -> (x+1=w23:T7)
  }
  n100 = call <vilib>:"Simple Error Handler.vi"("error in (no error)"=w11) -> ("error out"=→"error out":errorcluster)  [unwired: 4 in, 4 out]
